vi "Main.vi"(11 "Module Admin":refnum<class "Delacor_lib_QMH_Module Admin.lvclass">) -> ()   [LabVIEW 2020, in "CML UI.lvlib"]
doc: "This template is based off of the Queued Message Handler design pattern and the Queued Message Handler project template that ships with LabVIEW.\n\nThe main difference is that the queue is private to this module and communication between modules is performed via Broadcast and Request events.\n\nRequest events are wrapped in public API methods and are handled in the Event Handling Loop (EHL) of this VI. Any module can register for Broadcast events sent by this module. The EHL generates messages based on user interface actions.\n\nThe Message Handling Loop (MHL) processes messages generated by the EHL, or by other messages. The messages are string values, so new messages can be added easily to the Message Cases case structure in the MHL. Each message cluster can also provide an optional value for Message Data, which is a variant that can be converted to whatever message-specific data is required.\n_____\nBased on Delacor QMH Project Template 4.0.0.47.\n_____\nBased on DQMH Project Template 6.0.0.91."
uses:
  CML UI.lvlib
  <vilib>/Delacor/Delacor QMH/Libraries/Module Admin_class/Delacor_lib_QMH_Module Admin.lvclass
  Module Data--cluster.ctl
  Stop Argument--cluster.ctl
  <vilib>/Delacor/Delacor QMH/Libraries/Message Queue_class/Delacor_lib_QMH_Message Queue.lvclass/Delacor_lib_QMH_Message Queue.ctl
  <vilib>/Delacor/Delacor QMH/Libraries/Module Admin_class/Delacor_lib_QMH_Module Admin.lvclass/Delacor_lib_QMH_Module Admin.ctl
  <vilib>/Delacor/Delacor QMH/Libraries/Message Queue_class/Delacor_lib_QMH_Enqueue Message (Single).vi
  <vilib>/Delacor/Delacor QMH/Libraries/Module Admin_class/Delacor_lib_QMH_Get External Launch.vi
  <vilib>/Utility/error.llb/Error Cluster From Error Code.vi
  <vilib>/ErrorRing/Error Ring.xnode
  <vilib>/Delacor/Delacor QMH/Libraries/Message Queue_class/Delacor_lib_QMH_Message Queue.lvclass
  Settings Editor/Settings Editor.lvlib
  Acquisition/Acquisition.lvlib
  Logger/Logger.lvlib
panel:
  out "Logger Running?":bool
  out "Settings Editor Running?":bool
  out "Acquisition Running?":bool
  out "Data":waveform(dbl)[](graph)
  in  "Start Logging":bool
  out "Calibrated?":bool
  in  "Calibrate":bool
  in  "Settings":bool
  in  "Start":bool
  in  "Stop":bool
  out "error out":errorcluster
  out "Status":string
  out "version":string
  # "Continuous Measurement Data Logger"
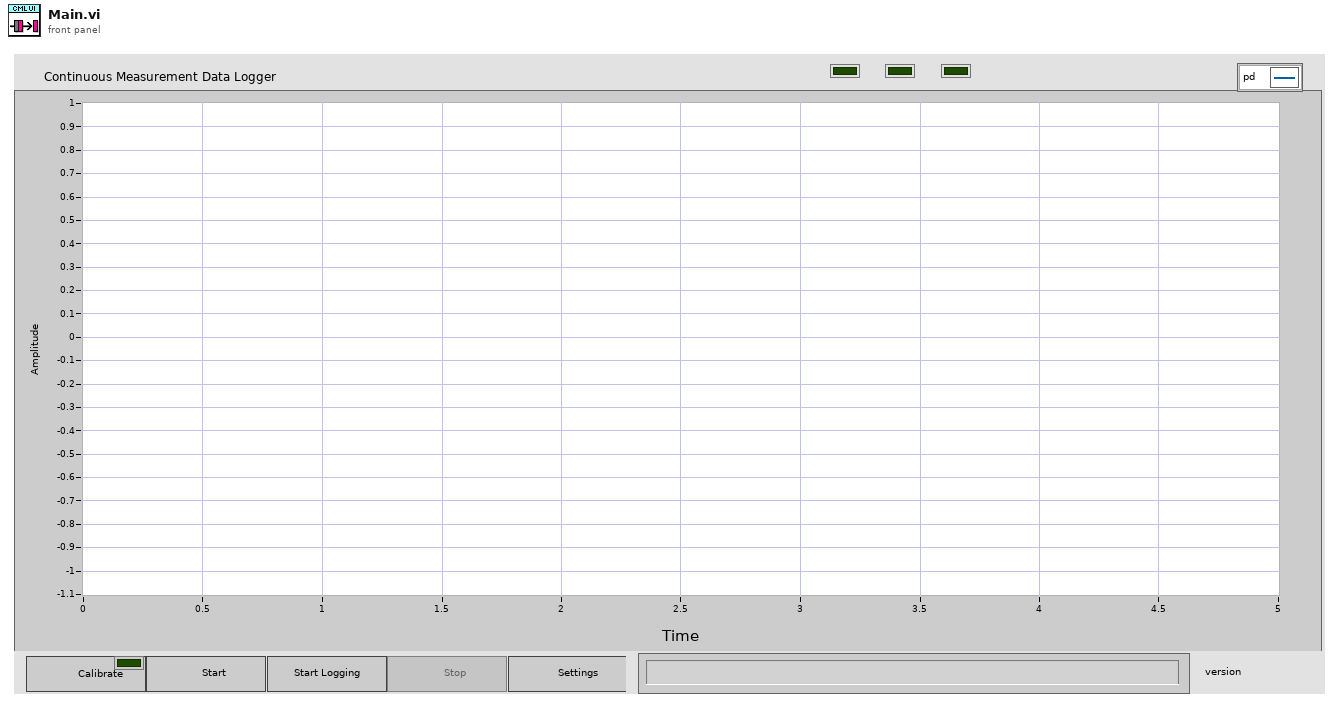
[diagram p1: front panel]
types:
  T1 = typedef "CML UI.lvlib/Request Events--cluster.ctl" = cluster{"Stop Module":refnum<user-event>, "Show Panel":refnum<user-event>, "Hide Panel":refnum<user-event>, "Get Module Execution Status":refnum<user-event>, "Show Diagram":refnum<user-event>}
  T2 = typedef "Settings Editor.lvlib/Broadcast Events--cluster.ctl" = cluster{"Module Did Init":refnum<user-event>, "Status Updated":refnum<user-event>, "Error Reported":refnum<user-event>, "Module Did Stop":refnum<user-event>, "Update Module Execution Status":refnum<user-event>, "Application Settings Updated":refnum<user-event>}
  T3 = typedef "Acquisition.lvlib/Broadcast Events--cluster.ctl" = cluster{"Module Did Init":refnum<user-event>, "Status Updated":refnum<user-event>, "Error Reported":refnum<user-event>, "Module Did Stop":refnum<user-event>, "Update Module Execution Status":refnum<user-event>, "Acquisition Started":refnum<user-event>, "Acquisition Stopped":refnum<user-event>, "Data Updated":refnum<user-event>, "Device Calibrated":refnum<user-event>}
  T4 = typedef "Logger.lvlib/Broadcast Events--cluster.ctl" = cluster{"Module Did Init":refnum<user-event>, "Status Updated":refnum<user-event>, "Error Reported":refnum<user-event>, "Module Did Stop":refnum<user-event>, "Update Module Execution Status":refnum<user-event>, "Logging Stopped":refnum<user-event>, "File Initialized":refnum<user-event>, "Logging Started":refnum<user-event>}
  T5 = typedef "CML UI.lvlib/Module Data--cluster.ctl" = cluster{"Status":string, "Measurement UI Controls":cluster{"Start Ref":refnum<vi>, "Stop Ref":refnum<vi>, "Settings Ref":refnum<vi>, "Status Ref":refnum<vi>, "Data Ref":refnum<vi>}}
  T6 = enum32{"invalid lock state", "Not Locked", "Locked (No Password)", "Password-protected"}
  T7 = typedef "CML UI.lvlib/Stop Argument--cluster.ctl" = cluster{"Origin":string, "Exit via Stop Module Req?":bool, "Wait for Module to stop?":bool}
  T8 = enum32{"Invalid", "Standard", "Closed", "Hidden", "Minimized", "Maximized"}
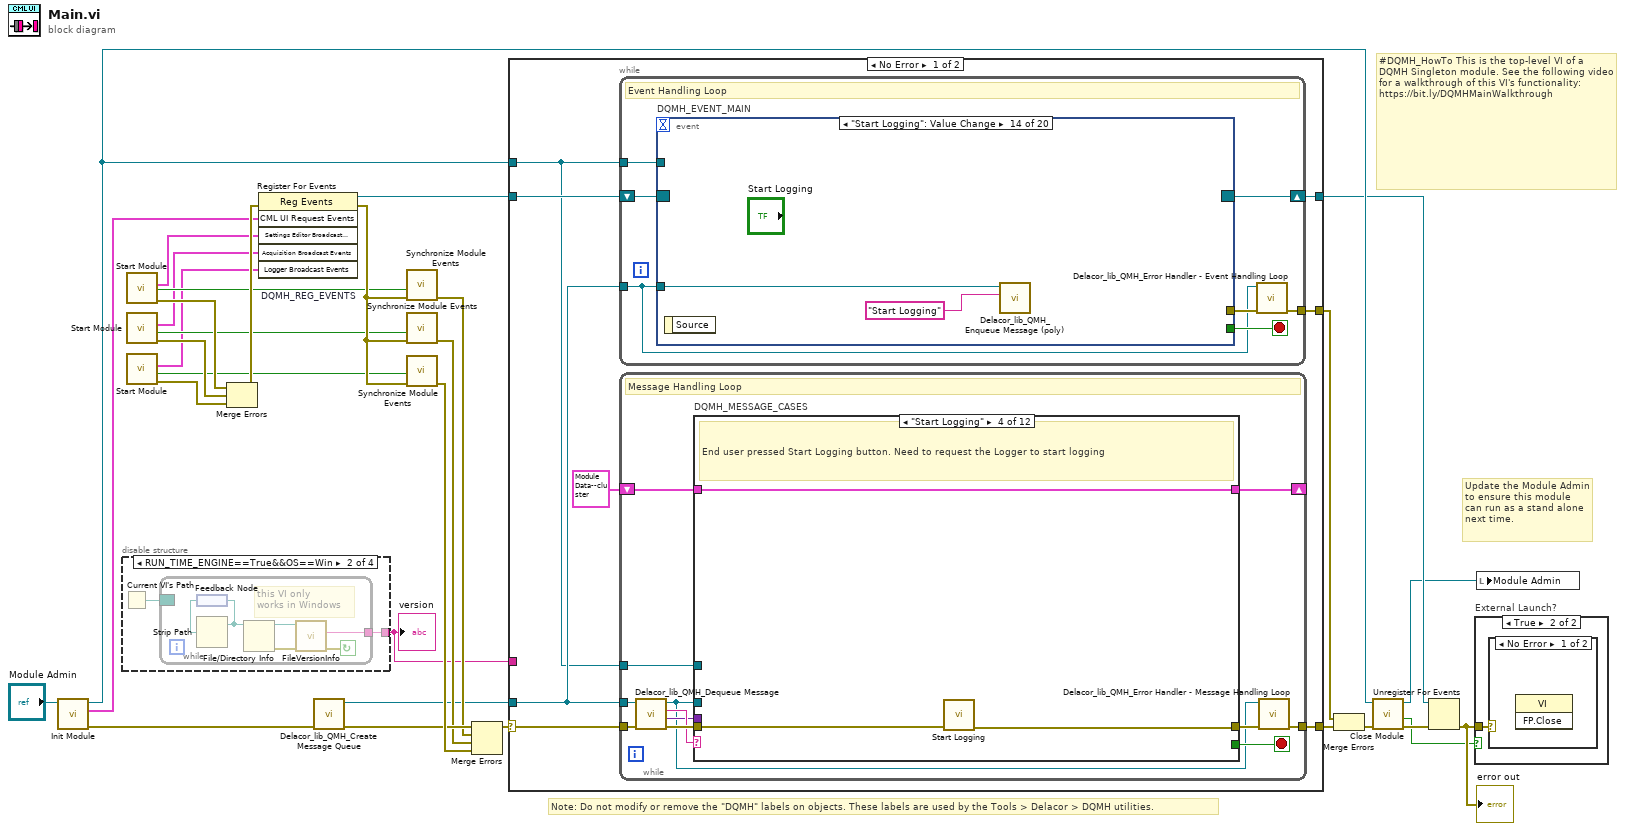
[diagram p0: block diagram]
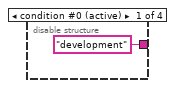
[diagram p2: hidden frame]
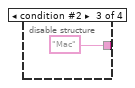
[diagram p3: hidden frame]
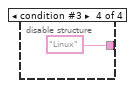
[diagram p4: hidden frame]
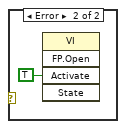
[diagram p6: hidden frame]
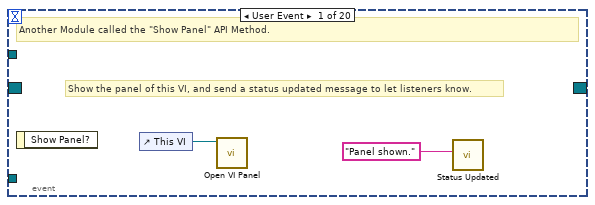
[diagram p7: hidden frame]
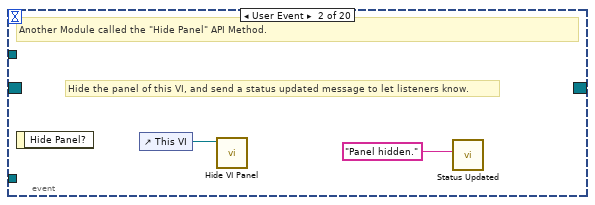
[diagram p8: hidden frame]
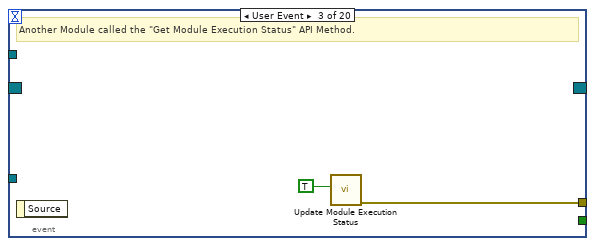
[diagram p9: hidden frame]
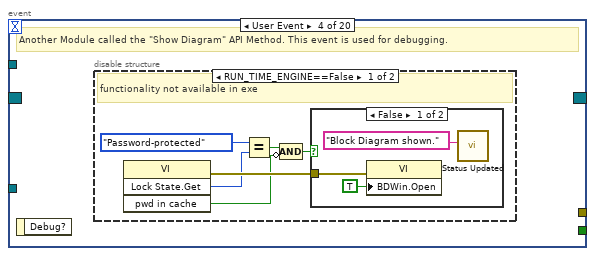
[diagram p10: hidden frame]
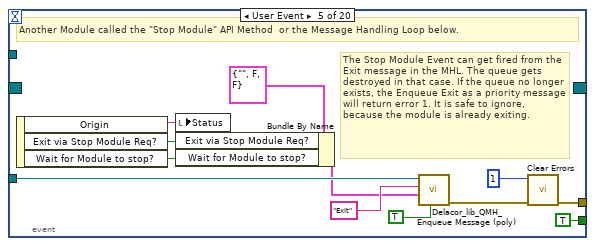
[diagram p13: hidden frame]
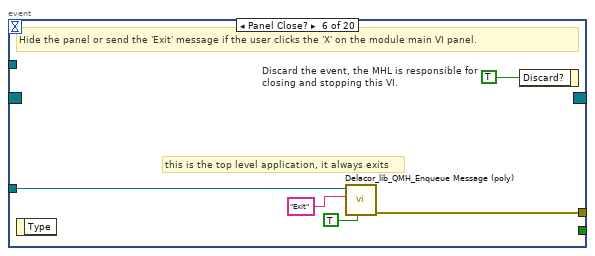
[diagram p14: hidden frame]
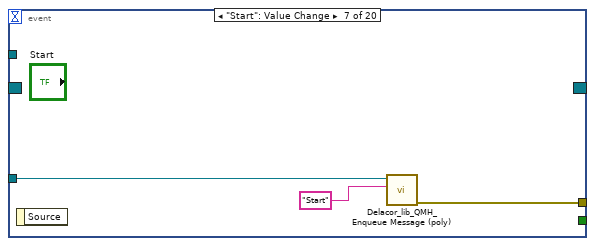
[diagram p15: hidden frame]
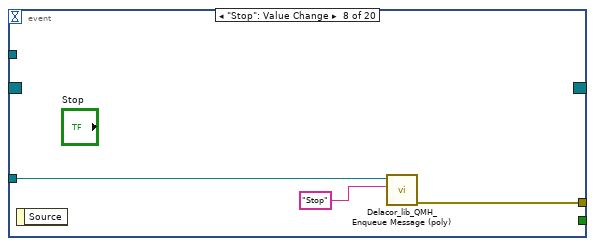
[diagram p16: hidden frame]
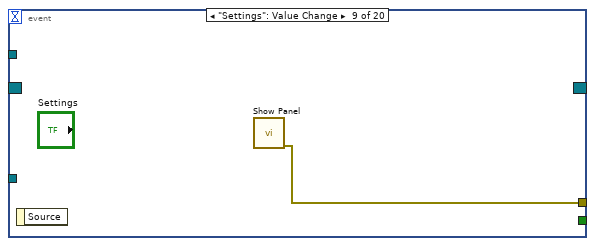
[diagram p17: hidden frame]
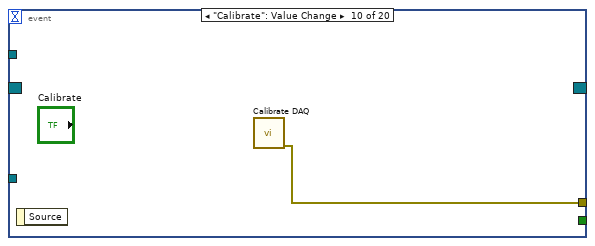
[diagram p18: hidden frame]
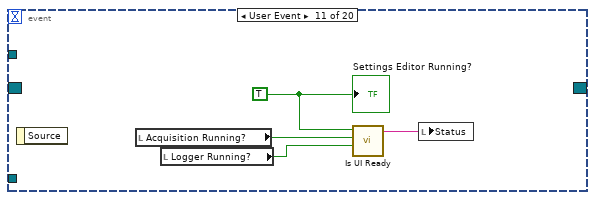
[diagram p19: hidden frame]
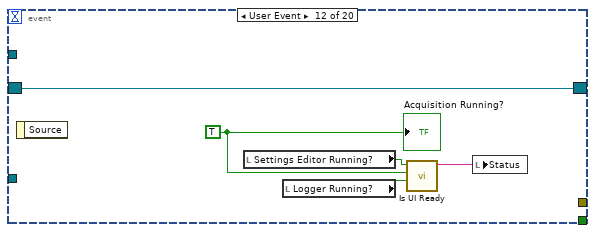
[diagram p20: hidden frame]
diagram:
  # "#DQMH_HowTo This is the top-level VI of a DQMH Singleton module. See the following video for a walkthrough of this VI's functionality: https://bit.ly/DQMHMainWalkthrough"
  # "Note: Do not modify or remove the \"DQMH\" labels on objects. These labels are used by the Tools > Delacor > DQMH utilities."
  # "Update the Module Admin to ensure this module can run as a stand alone next time."
  n1 = call "Init Module.vi"("Singleton Module Admin in"="Module Admin") -> ("error out"=w29:errorcluster, "CML UI Request Events"=w12:T1, "Singleton Module Admin out"=w15:refnum<class "Delacor_lib_QMH_Module Admin.lvclass">)  [unwired: 8 in]
  n2 = disable-structure "Conditional Disable Structure" shown="RUN_TIME_ENGINE==True&&OS==Win" {
    disable-tunnel: ["development" w33 "Mac" "Linux"] -> w1
    frame condition #0 (active) {
    }
    frame condition #1 {
      n3 = Current VI's Path() -> (path=w34:path)
      n4 = while {
        border: w34 -> [_]
        tunnel: [w35] -> w33
        stop <- w39 continue-if-true
        # "this VI only \nworks in Windows"
        n5 = feedback #1() -> (w38:path)
        n6 = Strip Path(path=w38) -> (stripped path=w37:path)  [unwired: 1 out]
        n7 = feedback-in #1(w37) -> ()
        n8 = File/Directory Info(path=w37) -> (path out=w36:path, error out=w40:errorcluster)  [unwired: 1 in, 5 out]
        n9 = call <vilib>:"FileVersionInfo.vi"("error in (no error)"=w40, "Application Path in"=w36) -> ("error out"=w39:errorcluster, "File Version Info"=w35:string)  [unwired: 6 in, 2 out]
      }
    }
    frame condition #2 {
    }
    frame condition #3 {
    }
  }
  "version" <- w1
  n10 = call "Start Module.vi"() -> ("error out"=w20:errorcluster, "Wait for Event Sync?"=w7:bool, "Settings Editor Broadcast Events"=w6:T2)  [unwired: 8 in, 1 out]
  n11 = call "Start Module.vi"() -> ("error out"=w19:errorcluster, "Wait for Event Sync?"=w4:bool, "Acquisition Broadcast Events"=w5:T3)  [unwired: 8 in, 1 out]
  n12 = call "Start Module.vi"() -> ("error out"=w18:errorcluster, "Wait for Event Sync?"=w2:bool, "Logger Broadcast Events"=w3:T4)  [unwired: 8 in, 1 out]
  n13 = Merge Errors(w20, w19, w18) -> (w17:errorcluster)
  n14 = register-events "DQMH_REG_EVENTS"(error in=w17, w12, w6, w5, w3) -> (reference out=w13:refnum<event-registration>, error out=w16:errorcluster)  [unwired: 1 in]
  n15 = call <vilib>:"Delacor_lib_QMH_Create Message Queue.vi"("error in"=w29) -> ("error out"=w24:errorcluster, "Message Queue"=w11:refnum<class "Delacor_lib_QMH_Message Queue.lvclass">)  [unwired: 9 in]
  n16 = call "Synchronize Module Events.vi"("error in (no error)"=w16, "Wait for Event Sync?"=w7) -> ("error out"=w22:errorcluster)  [unwired: 9 in]
  n17 = call "Synchronize Module Events.vi"("error in (no error)"=w16, "Wait for Event Sync?"=w4) -> ("error out"=w21:errorcluster)  [unwired: 9 in]
  n18 = call "Synchronize Module Events.vi"("error in (no error)"=w16, "Wait for Event Sync?"=w2) -> ("error out"=w31:errorcluster)  [unwired: 9 in]
  n19 = Merge Errors(w24, w22, w21, w31) -> (w23:errorcluster)
  n20 = case shown="No Error" w23 {
    selector: w23 -> [w48 w258]
    tunnel: [w50 w257] -> w30
    tunnel: [w47 w266] -> w14
    tunnel: w13 -> [w45 w266]
    tunnel: w11 -> [w44 w259]
    tunnel: [w49 _] -> w27
    tunnel: w15 -> [w43 w262]
    tunnel: w1 -> [_ _]
    frame No Error {
      n21 = while {
        tunnel: w44 -> [w51]
        shift-right: [w54] -> w47
        shift-left: w45 -> [w55]
        tunnel: [w56] -> w49
        tunnel: w43 -> [w52]
        stop <- w53 stop-if-true
        # "Event Handling Loop"
        n22 = event "DQMH_EVENT_MAIN" shown="[13] \"Start Logging\": Value Change" {
          selector: w55 -> [_ _ _ _ _ _ _ _ _ _ _ w106 _ _ _ _ _ _ _ _]
          dyn-events: [_ _ _ _ _ _ _ _ _ _ _ w106 _ _ _ _ _ _ _ _] -> w54
          timeout: _ -> [_ _ _ _ _ _ _ _ _ _ _ _ _ _ _ _ _ _ _ _]
          tunnel: [_ _ _ _ TRUE ("Discard?") _ _ _ _ _ _ _ _ _ _ _ _ _ _ _] -> w53
          tunnel: w51 -> [_ _ _ _ w80 w87 w90 w93 _ _ _ _ _ w111 _ _ w120 w122 _ _]
          tunnel: [_ _ w63 _ w83 w89 w92 w95 w96 w97 _ _ _ _ _ w118 _ _ _ _] -> w57
          tunnel: w52 -> [_ _ _ _ _ _ _ _ _ _ _ _ _ _ _ _ _ _ _ _]
          event User Event {
            # "Show the panel of this VI, and send a status updated message to let listeners know."
            # "Another Module called the \"Show Panel\" API Method."
            n23 = event-data() -> ()  [unwired: 1 in, 1 out]
            n24 = control-ref of="This VI"() -> (w59:refnum<vi>)
            n25 = call "Open VI Panel.vi"("VI"=w59) -> ()  [unwired: 10 in, 1 out]
            n26 = call "Status Updated.vi"("Status"="Panel shown." ("format string")) -> ()  [unwired: 10 in, 1 out]
          }
          event User Event {
            # "Hide the panel of this VI, and send a status updated message to let listeners know."
            # "Another Module called the \"Hide Panel\" API Method."
            n27 = event-data() -> ()  [unwired: 1 in, 1 out]
            n28 = control-ref of="This VI"() -> (w61:refnum<vi>)
            n29 = call "Hide VI Panel.vi"("VI"=w61) -> ()  [unwired: 10 in, 1 out]
            n30 = call "Status Updated.vi"("Status"="Panel hidden." ("format string")) -> ()  [unwired: 10 in, 1 out]
          }
          event User Event {
            # "Another Module called the \"Get Module Execution Status\" API Method."
            n31 = event-data() -> ()  [unwired: 1 in, 1 out]
            n32 = call "Update Module Execution Status.vi"("Running?"=TRUE) -> ("error out"=w63:errorcluster)  [unwired: 10 in]
          }
          event User Event {
            # "Another Module called the \"Show Diagram\" API Method. This event is used for debugging."
            n33 = event-data() -> ()  [unwired: 1 in, 1 out]
            n34 = disable-structure shown="RUN_TIME_ENGINE==False" {
              frame condition #0 (active) {
                # "functionality not available in exe"
                n35 = invoke on="Invoke Node" class="VI" method="Lock State.Get"() -> (error out=w69:errorcluster, "Get Lock State"=w68:T6, "pwd in cache"=w65:bool)  [unwired: 4 in, 1 out]
                n36 = Equal?(x=T6."Password-protected", y=w68) -> (x = y?=w66:bool)
                n37 = Compound Arithmetic op=AND(w66, invert w65) -> (w64:bool)
                n38 = case shown="False" w64 {
                  tunnel: w69 -> [w72 _]
                  frame False {
                    n39 = property on="Property Node" class="VI"(error in=w72, "BDWin.Open"=TRUE ("Block Diagram Window:Open")) -> ()  [unwired: 1 in, 2 out]
                    n40 = call "Status Updated.vi"("Status"="Block Diagram shown." ("format string")) -> ()  [unwired: 10 in, 1 out]
                  }
                  frame True {
                    # "Password-protected VI, and the password is not in the cache. Do not show the diagram."
                  }
                }
              }
              frame condition #1 {
              }
            }
          }
          event User Event {
            # "The Stop Module Event can get fired from the Exit message in the MHL. The queue gets destroyed in that case. If the queue no longer exists, the Enqueue Exit as a priority message will return error 1. It is safe to ignore, because the module is already exiting."
            # "Another Module called the \"Stop Module\" API Method  or the Message Handling Loop below."
            n41 = event-data() -> ("Origin"=w79:string, "Exit via Stop Module Req?"=w75:bool, "Wait for Module to stop?"=w74:bool)  [unwired: 1 in]
            n42 = local write "Status"(w79) -> ()
            n43 = Bundle By Name(cluster=T7 {"Origin"="", "Exit via Stop Module Req?"=FALSE, "Wait for Module to stop?"=FALSE} ("Stop Argument"), "Exit via Stop Module Req?"=w75, "Wait for Module to stop?"=w74) -> (w73:T7)
            n44 = call-poly <vilib>:"Delacor_lib_QMH_Enqueue Message (poly).vi"("Priority Message? (F)"=TRUE, "Message Data"=w73, "Message"="Exit", "Message Queue in"=w80) -> ("error out"=w84:errorcluster)  [unwired: 6 in, 1 out]
            n45 = call <vilib>:"Clear Errors.vi"("error in (no error)"=w84, "specific error code to clear (0: all)"=1) -> ("error out"=w83:errorcluster)  [unwired: 4 in, 1 out]
          }
          event Panel Close? {
            w88 = TRUE  # Discard the event, the MHL is responsible for closing and stopping this VI.
            # "this is the top level application, it always exits"
            # "Hide the panel or send the 'Exit' message if the user clicks the 'X' on the module main VI panel."
            n46 = event-data() -> ()  [unwired: 1 in, 1 out]
            n47 = call-poly <vilib>:"Delacor_lib_QMH_Enqueue Message (poly).vi"("Priority Message? (F)"=TRUE, "Message"="Exit", "Message Queue in"=w87) -> ("error out"=w89:errorcluster)  [unwired: 7 in, 1 out]
            n48 = event-data ("Event Filter Node")("Discard?"=w88) -> ()  [unwired: 1 in, 1 out]
          }
          event "Start": Value Change {
            n49 = event-data() -> ()  [unwired: 1 in, 1 out]
            n50 = call-poly <vilib>:"Delacor_lib_QMH_Enqueue Message (poly).vi"("Message"="Start", "Message Queue in"=w90) -> ("error out"=w92:errorcluster)  [unwired: 8 in, 1 out]
          }
          event "Stop": Value Change {
            n51 = event-data() -> ()  [unwired: 1 in, 1 out]
            n52 = call-poly <vilib>:"Delacor_lib_QMH_Enqueue Message (poly).vi"("Message"="Stop", "Message Queue in"=w93) -> ("error out"=w95:errorcluster)  [unwired: 8 in, 1 out]
          }
          event "Settings": Value Change {
            n53 = event-data() -> ()  [unwired: 1 in, 1 out]
            n54 = call "Show Panel.vi"() -> ("error out"=w96:errorcluster)  [unwired: 11 in]
          }
          event "Calibrate": Value Change {
            n55 = event-data() -> ()  [unwired: 1 in, 1 out]
            n56 = call "Calibrate DAQ.vi"() -> ("error out"=w97:errorcluster)  [unwired: 11 in]
          }
          event User Event {
            w99 = TRUE ("Settings Editor Running?")
            n57 = event-data() -> ()  [unwired: 1 in, 1 out]
            n58 = local read "Acquisition Running?"() -> (w101:bool)
            n59 = local read "Logger Running?"() -> (w100:bool)
            n60 = call "Is UI Ready.vi"("Logger Running?"=w100, "Acquisition Running?"=w101, "Settings Editor Running?"=w99) -> ("Status"=w98:string)  [unwired: 8 in]
            n61 = local write "Status"(w98) -> ()
            "Settings Editor Running?" <- w99
          }
          event User Event {
            w104 = TRUE ("Acquisition Running?")
            n62 = event-data() -> ()  [unwired: 1 in, 1 out]
            n63 = local read "Settings Editor Running?"() -> (w103:bool)
            n64 = local read "Logger Running?"() -> (w102:bool)
            n65 = call "Is UI Ready.vi"("Logger Running?"=w102, "Acquisition Running?"=w104, "Settings Editor Running?"=w103) -> ("Status"=w105:string)  [unwired: 8 in]
            n66 = local write "Status"(w105) -> ()
            "Acquisition Running?" <- w104
          }
          event User Event {
            w109 = TRUE ("Logger Running?")
            n67 = event-data() -> ()  [unwired: 1 in, 1 out]
            n68 = local read "Settings Editor Running?"() -> (w108:bool)
            n69 = local read "Acquisition Running?"() -> (w107:bool)
            n70 = call "Is UI Ready.vi"("Logger Running?"=w109, "Acquisition Running?"=w107, "Settings Editor Running?"=w108) -> ("Status"=w110:string)  [unwired: 8 in]
            n71 = local write "Status"(w110) -> ()
            "Logger Running?" <- w109
          }
          event "Start Logging": Value Change {
            n72 = event-data() -> ()  [unwired: 1 in, 1 out]
            n73 = call-poly <vilib>:"Delacor_lib_QMH_Enqueue Message (poly).vi"("Message"="Start Logging", "Message Queue in"=w111) -> ()  [unwired: 8 in, 2 out]
          }
          event User Event {
            n74 = event-data() -> ("Status"=w113:string)  [unwired: 1 in]
            "Status" <- w113
            n75 = call "Status Updated.vi"("Status"=w113) -> ()  [unwired: 10 in, 1 out]
          }
          event User Event {
            n76 = event-data() -> ("Error"=w118:errorcluster, "Module Name"=w116:string)  [unwired: 1 in, 1 out]
            n77 = Unbundle By Name(w118) -> ("code"=w117:i32)
            n78 = Format Into String(format string="Error %d at %s", w117, w116) -> (resulting string=w115:string)  [unwired: 2 in, 1 out]
            n79 = local write "Status"(w115) -> ()
          }
          event User Event {
            n80 = event-data() -> ()  [unwired: 1 in, 1 out]
            n81 = call-poly <vilib>:"Delacor_lib_QMH_Enqueue Message (poly).vi"("Message"="Acquisition Started Interlocks", "Message Queue in"=w120) -> ()  [unwired: 8 in, 2 out]
          }
          event User Event {
            n82 = event-data() -> ()  [unwired: 1 in, 1 out]
            n83 = call-poly <vilib>:"Delacor_lib_QMH_Enqueue Message (poly).vi"("Message"="Acquisition Stopped Interlocks", "Message Queue in"=w122) -> ()  [unwired: 8 in, 2 out]
          }
          event User Event {
            n84 = event-data() -> ("Graph Data"=→"Data":waveform(dbl)[])  [unwired: 1 in]
          }
          event User Event {
            n85 = event-data() -> ()  [unwired: 1 in, 1 out]
            "Calibrated?" <- TRUE ("Calibrated?")
          }
        }
        n86 = call-dynamic "Delacor_lib_QMH_Error Handler - Event Handling Loop.vi"("error in"=w57, "Message Queue in"=w51) -> ("dup error in"=w56:errorcluster)  [unwired: 8 in, 1 out]
      }
      n87 = while {
        tunnel: w44 -> [w127]
        shift-right: [w131] -> _
        shift-left: T5 {"Status"="", "Measurement UI Controls"={"Start Ref"=refnum, "Stop Ref"=refnum, "Settings Ref"=refnum, "Status Ref"=refnum, "Data Ref"=refnum}} ("Data Cluster") -> [w132]
        tunnel: w48 -> [w135]
        tunnel: [w133] -> w50
        tunnel: w43 -> [w125]
        stop <- w130 stop-if-true
        # "Message Handling Loop"
        n88 = call-dynamic "Delacor_lib_QMH_Dequeue Message.vi"("error in"=w135, "Message Queue in"=w127) -> ("error out"=w134:errorcluster, "Message Data"=w128:variant, "Message"=w129:string, "Message Queue out"=w126:refnum<class "Delacor_lib_QMH_Message Queue.lvclass">)  [unwired: 6 in]
        n89 = case "DQMH_MESSAGE_CASES" shown="\"Start Logging\"" w129 {
          selector: w129 -> [_ _ _ _ _ _ _ _ _ _ _ w244]
          tunnel: w126 -> [_ _ _ _ _ _ _ _ _ w208 w235 _]
          tunnel: w134 -> [w167 w171 w174 w177 w187 w190 w200 w203 w205 w215 w240 w246]
          tunnel: [w165 w171 w173 w176 w187 w189 w200 w202 w205 w211 w224 w247] -> w136
          tunnel: w132 -> [w156 w170 w172 w178 w179 w188 w192 w201 w204 w210 w234 w245]
          tunnel: [w145 w170 w172 w178 w179 w188 w192 w201 w204 w210 w234 w245] -> w131
          tunnel: [_ _ _ _ _ _ _ _ _ _ w233 _] -> w130
          tunnel: w128 -> [_ _ _ _ _ _ _ _ _ w209 w232 _]
          tunnel: w125 -> [w157 _ _ _ _ _ _ _ _ w207 w227 _]
          frame "Initialize" {
            w151 = "Initial Message" ("Initial Message")
            # "Enable: Start, Settings\nDisable: Stop"
            # "Initialize - Any operation that needs to be done before the module can receive messages. Synchronize Caller Events.vi will inform Start Module.vi that the module has launched and is ready to receive messages. Module Did Init.vi will broadcast that the module initialized."
            n90 = call "Synchronize Caller Events.vi"("error in (no error)"=w167, "Singleton Module Admin in"=w157) -> ("error out"=w166:errorcluster, "Singleton Module Admin out"=w153:refnum<class "Delacor_lib_QMH_Module Admin.lvclass">)  [unwired: 8 in]
            n91 = property on="Property Node" class="Module Admin"(reference=w153) -> ("Accessors:External Launch"=w161:bool)  [unwired: 1 in, 2 out]
            n92 = property on="Data" class="WFChart (strict)"("History Data"=waveform(dbl)[][] []) -> ()  [unwired: 2 in, 2 out]
            n93 = control-ref of="Data"() -> (w146:refnum<vi>)
            n94 = local write "Calibrated?"(FALSE ("Calibrated?")) -> ()
            n95 = control-ref of="Start"() -> (w150:refnum<vi>)
            n96 = control-ref of="Stop"() -> (w149:refnum<vi>)
            n97 = control-ref of="Settings"() -> (w148:refnum<vi>)
            n98 = control-ref of="Status"() -> (w147:refnum<vi>)
            n99 = Select(t=T8."Hidden" ("State"), s=w161, f=T8."Standard" ("State")) -> (s? t:f=w158:T8)
            n100 = call "Module Name--constant.vi"() -> ("Module Name"=w164:string)  [unwired: 11 in]
            n101 = Bundle By Name(cluster=w156, "Measurement UI Controls.Start Ref"=w150, "Measurement UI Controls.Stop Ref"=w149, "Measurement UI Controls.Settings Ref"=w148, "Measurement UI Controls.Status Ref"=w147, "Measurement UI Controls.Data Ref"=w146, "Status"=w151) -> (w145:T5)
            n102 = local write "Status"(w151) -> ()
            n103 = property on="Property Node" class="VI"("Front Panel.Title"=w164) -> (reference out=w163:refnum<vi>, error out=w169:errorcluster)  [unwired: 2 in]
            n104 = invoke on="Invoke Node" class="VI" method="FP.Open"(reference=w163, error in=w169, "State"=w158) -> (reference out=w162:refnum<vi>, error out=w168:errorcluster)  [unwired: 2 in, 3 out]
            n105 = Unbundle By Name(w145) -> ("Measurement UI Controls.Start Ref"=w144:refnum<vi>, "Measurement UI Controls.Settings Ref"=w143:refnum<vi>, "Measurement UI Controls.Stop Ref"=w140:refnum<vi>)
            n106 = call "Module Name--constant.vi"() -> ("Module Name"=w154:string)  [unwired: 11 in]
            n107 = invoke on="Invoke Node" class="VI" method="FP.Center"(reference=w162, error in=w168) -> ()  [unwired: 1 in, 3 out]
            n108 = Build Array(w144, w143) -> (w142:refnum<vi>[])
            n109 = Build Array(w140) -> (w139:refnum<vi>[])
            n110 = call "Module Did Init.vi"("error in (no error)"=w166, "Initialized?"=TRUE, "Origin"=w154) -> ("error out"=w165:errorcluster)  [unwired: 8 in]
            n111 = call "Set Enable State on Multiple Controls.vi"("Enable?"=FALSE, "Controls"=w139) -> ()  [unwired: 10 in]
            n112 = call "Set Enable State on Multiple Controls.vi"("Enable?"=TRUE, "Controls"=w142) -> ()  [unwired: 10 in]
          }
          frame "---Module Specific---" {
            # "Separator -- The following cases handle messages specific to this Module."
          }
          frame "Start" {
            # "End user pressed Start button. Need to request for Acquisition to start acquiring and for initialize file for logging"
            n113 = call "Initialize File.vi"("error in (no error)"=w174) -> ("error out"=w175:errorcluster)  [unwired: 8 in, 2 out]
            n114 = call "Start Acquiring.vi"("error in (no error)"=w175) -> ("error out"=w173:errorcluster)  [unwired: 8 in, 2 out]
          }
          frame "Start Logging" {
            # "End user pressed Start Logging button. Need to request the Logger to start logging"
            n115 = call "Start Logging.vi"("error in"=w177) -> ("error out"=w176:errorcluster)  [unwired: 10 in]
          }
          frame "Acquisition Started Interlocks" {
            # "Enable: Stop\nDisable: Start, Settings"
            n116 = Unbundle By Name(w179) -> ("Measurement UI Controls.Stop Ref"=w186:refnum<vi>, "Measurement UI Controls.Start Ref"=w181:refnum<vi>, "Measurement UI Controls.Settings Ref"=w180:refnum<vi>)
            n117 = Build Array(w186) -> (w185:refnum<vi>[])
            n118 = Build Array(w181, w180) -> (w182:refnum<vi>[])
            n119 = call "Set Enable State on Multiple Controls.vi"("Enable?"=TRUE, "Controls"=w185) -> ()  [unwired: 10 in]
            n120 = call "Set Enable State on Multiple Controls.vi"("Enable?"=FALSE, "Controls"=w182) -> ()  [unwired: 10 in]
          }
          frame "Stop" {
            # "End user pressed Stop button. Need to request for Acquisition to stop acquiring and for Logger to stop logging."
            n121 = call "Stop Acquiring.vi"("error in (no error)"=w190) -> ("error out"=w191:errorcluster)  [unwired: 10 in]
            n122 = call "Stop Logging.vi"("error in (no error)"=w191) -> ("error out"=w189:errorcluster)  [unwired: 10 in]
          }
          frame "Acquisition Stopped Interlocks" {
            # "Enable: Start, Settings\nDisable: Stop"
            n123 = Unbundle By Name(w192) -> ("Measurement UI Controls.Stop Ref"=w197:refnum<vi>, "Measurement UI Controls.Start Ref"=w196:refnum<vi>, "Measurement UI Controls.Settings Ref"=w195:refnum<vi>)
            n124 = Build Array(w197) -> (w199:refnum<vi>[])
            n125 = Build Array(w196, w195) -> (w194:refnum<vi>[])
            n126 = call "Set Enable State on Multiple Controls.vi"("Enable?"=FALSE, "Controls"=w199) -> ()  [unwired: 10 in]
            n127 = call "Set Enable State on Multiple Controls.vi"("Enable?"=TRUE, "Controls"=w194) -> ()  [unwired: 10 in]
          }
          frame "---Copy This Frame---" {
            # "Duplicate this frame when creating new messages.  Change this comment in the duplicated frame to describe this message."
            n128 = Merge Errors(w203) -> (w202:errorcluster)
          }
          frame "---Exit and Error Handling---" {
            # "Separator - The following cases handle errors and exit messages."
          }
          frame "Error" {
            # "Error - Check the error message data and respond accordingly. This message is sent by the \"Error Handler\" VIs at the end of each loop in this application."
            n129 = property on="Property Node" class="Module Admin"(reference=w207) -> ("Accessors:External Launch"=w206:bool)  [unwired: 1 in, 2 out]
            n130 = Variant To Data(error in=w215, type=errorcluster {"status"=FALSE, "code"=0, "source"=""} ("error constant"), Variant=w209) -> (data=w216:errorcluster, error out=w213:errorcluster)
            n131 = call "Error Reported.vi"("Error"=w216) -> ()  [unwired: 10 in, 1 out]
            n132 = case shown="False" w206 {
              tunnel: [w221 _] -> w212
              tunnel: w208 -> [w219 _]
              tunnel: w216 -> [w220 _]
              frame False {
                # "If the module is running standalone, then pop up an error dialog and call the \"Exit\" message."
                n133 = call <vilib>:"Simple Error Handler.vi"("error in (no error)"=w220) -> ()  [unwired: 4 in, 5 out]
                n134 = call-poly <vilib>:"Delacor_lib_QMH_Enqueue Message (poly).vi"("Priority Message? (F)"=TRUE, "Message"="Exit", "Message Queue in"=w219) -> ("error out"=w221:errorcluster)  [unwired: 7 in, 1 out]
              }
              frame True {
                # "If the module was launched externally, calling the Error Reported broadcast VI is the only action performed by the \"Error\" message. The module's caller can then process the error appropriately."
              }
            }
            n135 = Merge Errors(w213, w212) -> (w211:errorcluster)
            n136 = local write "error out"(w211) -> ()
          }
          frame "Exit" {
            w226 = TRUE ("Wait for Module to Stop? (F)")
            w231 = 91  # 91: not all Exit messages will have an argument
            w233 = TRUE  # Stop the VI
            # "DAQ and LOG modules use the settings editor. CML UI module waits for both modules to completely stop before stopping the settings editor."
            # "Release the message queue reference"
            # "Exit - Exit the application."
            n137 = Variant To Data(error in=w240, type=T7 {"Origin"="", "Exit via Stop Module Req?"=FALSE, "Wait for Module to stop?"=FALSE} ("Stop Argument"), Variant=w232) -> (data=w229:T7, error out=w237:errorcluster)
            n138 = call <vilib>:"Clear Errors.vi"("error in (no error)"=w237, "specific error code to clear (0: all)"=w231) -> ("error out"=w239:errorcluster)  [unwired: 4 in, 1 out]
            n139 = control-ref of="This VI"() -> (w228:refnum<vi>)
            n140 = call "Module Name--constant.vi"() -> ("Module Name"=w225:string)  [unwired: 11 in]
            n141 = call "Handle Exit.vi"("Stop Argument"=w229, "Admin in"=w227, "VI reference"=w228) -> ("error out"=w236:errorcluster)  [unwired: 7 in, 1 out]
            n142 = call "Stop Module.vi"("Wait for Module to Stop? (F)"=w226, "Origin"=w225) -> ("error out"=w223:errorcluster)  [unwired: 9 in]
            n143 = call "Stop Module.vi"("Wait for Module to Stop? (F)"=w226, "Origin"=w225) -> ("error out"=w222:errorcluster)  [unwired: 9 in]
            n144 = call-dynamic "Delacor_lib_QMH_Release Message Queue.vi"("error in"=w239, "Message Queue"=w235) -> ("error out"=w238:errorcluster)  [unwired: 9 in]
            n145 = Merge Errors(w223, w222) -> (w241:errorcluster)
            n146 = Merge Errors(w238, w236) -> (w224:errorcluster)
            n147 = call <vilib>:"Clear Errors.vi"("error in (no error)"=w241) -> ("error out"=w242:errorcluster)  [unwired: 5 in, 1 out]
            n148 = call "Stop Module.vi"("error in (no error)"=w242, "Wait for Module to Stop? (F)"=w226, "Origin"=w225) -> ()  [unwired: 8 in, 1 out]
          }
          frame Default {
            # "'Default' case only runs if there is a message that isn't defined in any of the other cases.  Output a programming error."
            n149 = call "Module Name--constant.vi"() -> ("Module Name"=w243:string)  [unwired: 11 in]
            n150 = xnode ("Error Ring")("parameter 0"=w244, "parameter 1"=w243) -> ("error out"=w248:errorcluster)
            n151 = Merge Errors(w246, w248) -> (w247:errorcluster)
          }
        }
        n152 = call-dynamic "Delacor_lib_QMH_Error Handler - Message Handling Loop.vi"("error in"=w136, "Message Queue in"=w126) -> ("dup error in"=w133:errorcluster)  [unwired: 8 in, 1 out]
      }
    }
    frame Error {
      w261 = TRUE ("Wait for Module to Stop? (F)")
      # "Synchronize Caller Events.vi will inform Start Module.vi that the module has launched and will let the code calling Start Module.vi register for broadcasts and would permit the caller receive the broadcast that an error occurred at launch time."
      n153 = call-dynamic "Delacor_lib_QMH_Release Message Queue.vi"("error in"=w258, "Message Queue"=w259) -> ("error out"=w257:errorcluster)  [unwired: 9 in]
      n154 = call "Synchronize Caller Events.vi"("Singleton Module Admin in"=w262) -> ("error out"=w267:errorcluster)  [unwired: 9 in, 1 out]
      n155 = call "Module Name--constant.vi"() -> ("Module Name"=w265:string)  [unwired: 11 in]
      n156 = call "Module Name--constant.vi"() -> ("Module Name"=w260:string)  [unwired: 11 in]
      n157 = call "Stop Module.vi"("Wait for Module to Stop? (F)"=w261, "Origin"=w260) -> ()  [unwired: 9 in, 1 out]
      n158 = call "Stop Module.vi"("Wait for Module to Stop? (F)"=w261, "Origin"=w260) -> ()  [unwired: 9 in, 1 out]
      n159 = call "Stop Module.vi"("Wait for Module to Stop? (F)"=w261, "Origin"=w260) -> ()  [unwired: 9 in, 1 out]
      n160 = Format Into String(format string="An error occurred during initialization. %s is no longer running.", w265) -> (resulting string=w263:string)  [unwired: 2 in, 1 out]
      n161 = Merge Errors(w257, w267) -> (w268:errorcluster)
      n162 = call "Error Reported.vi"("Additional Information"=w263, "Error"=w268) -> ()  [unwired: 9 in, 1 out]
    }
  }
  n163 = Merge Errors(w27, w30) -> (w26:errorcluster)
  n164 = call "Close Module.vi"("error in (no error)"=w26, "Module Admin in"=w15) -> ("error out"=w28:errorcluster, "External Launch"=w8:bool, "Module Admin out"=w9:refnum<class "Delacor_lib_QMH_Module Admin.lvclass">)  [unwired: 7 in]
  n165 = Unregister For Events(event registration refnum=w14, error in=w28) -> (error out=w25:errorcluster)
  "error out" <- w25
  n166 = case "External Launch?" shown="True" w8 {
    tunnel: w25 -> [_ w269]
    frame False {
    }
    frame True {
      n167 = case shown="No Error" w269 {
        frame No Error {
          n168 = invoke class="VI" method="FP.Close"() -> ()  [unwired: 3 in, 3 out]
        }
        frame Error {
          n169 = invoke on="Invoke Node" class="VI" method="FP.Open"("Activate"=TRUE ("Activate?")) -> ()  [unwired: 4 in, 5 out]
        }
      }
    }
  }
  n170 = local write "Module Admin"(w9) -> ()
